vi "write.vi"() -> ()   [LabVIEW 2016]
uses:
  <vilib>/Instr/_visa.llb/VISA Configure Serial Port (Serial Instr).vi
panel:
  out "Numeric":dbl
  in  "Set Relay voltage":dbl(slide)=9.0 scale=0.0..10.0
  out "Compressor Status":bool
  out "Helium Underpressure":bool=TRUE
  in  "Pressure Lower Limit":dbl=0.1
  out "Helium Overpressure":bool
  in  "Pressure Upper Limit":dbl=2.8
  in  "Reading 2":string(combo)="255:R:OTEMP"
  out "Monitor 2":dbl(graph)
  out "Temperature":dbl=23.05
  in  "monitor 2 read length":u32=25
  out "monitor 2 feedback":string
  in  "Reading 1":string(combo)="255:R:MRMD"
  in  "Abort monitoring":bool
  out "Puressure":dbl=0.009
  in  "monitor 1 read length":u32=25
  out "Monitor 1":dbl(graph)
  out "Monitor 1 feedback":string
  # "psi"
  # "°C"
  # "Serial Port I/O control"
  # "Relay Configuration"
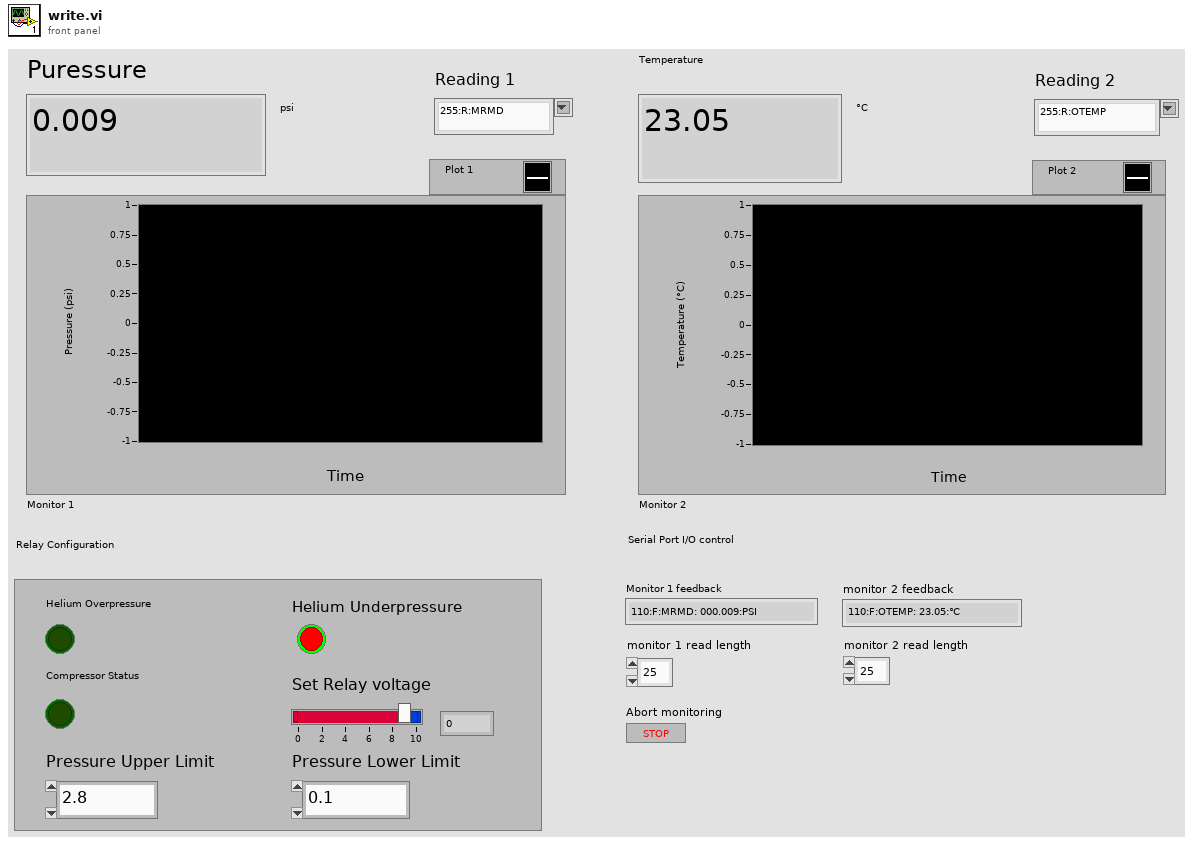
[diagram p1: front panel]
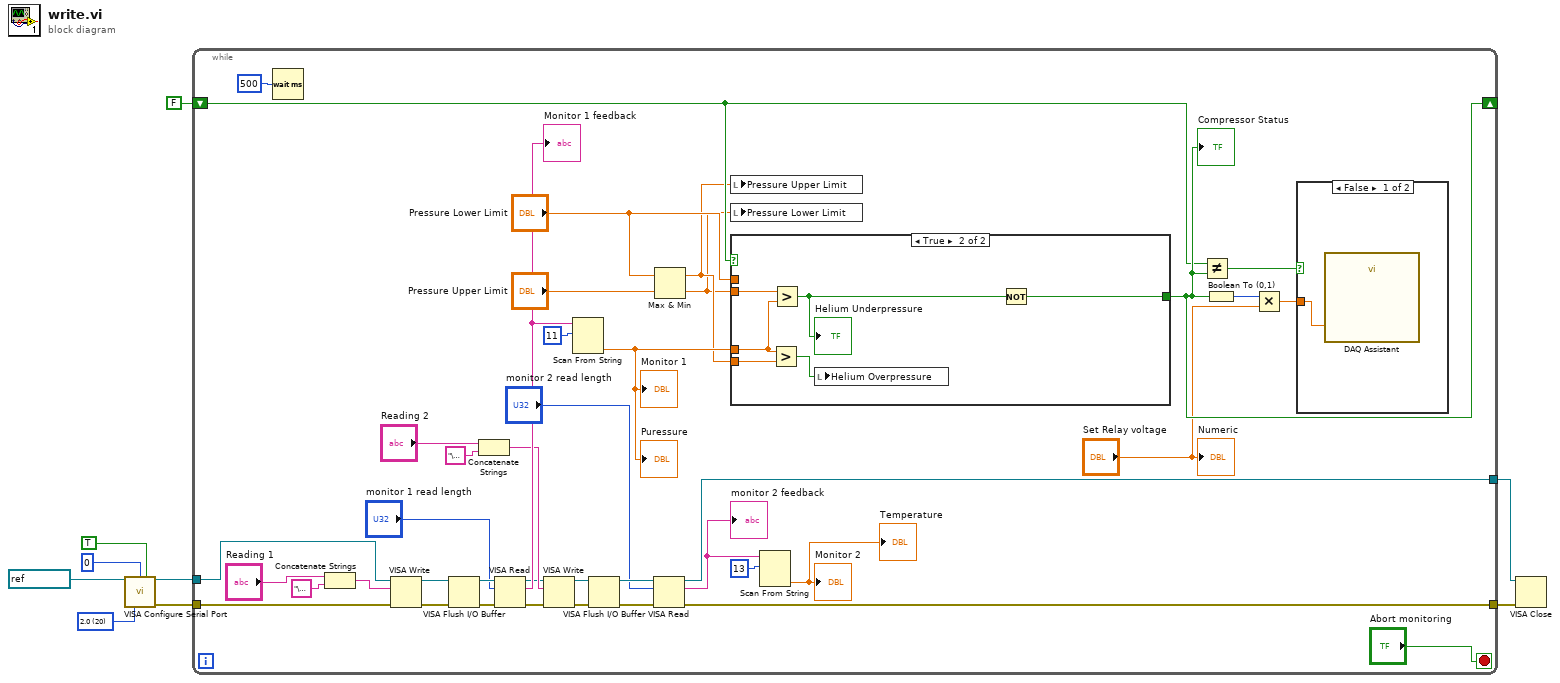
[diagram p0: block diagram]
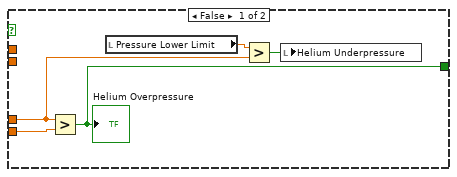
[diagram p3: hidden frame]
diagram:
  w4 = u16 20 items=["1.0"=10, "1.5"=15, "2.0"=20] ("stop bits (10: 1 bit)")
  n1 = call-poly "VISA Configure Serial Port"("VISA resource name"=refnum<visa-resource-name> "COM2", "termination char\n(0xA = '\\n' = LF)"=u8 0 ("termination char\n(0xA = '\\n' = LF)"), "Enable Termination\nChar (T)"=TRUE ("Enable Termination\nChar (T)"), "stop bits (10: 1 bit)"=w4) -> ("VISA resource name out"=w1:refnum<visa-resource-name>, "error out"=w3:errorcluster)  [unwired: 10 in]
  n2 = while {
    tunnel: [w23] -> w9
    tunnel: [w24] -> w8
    tunnel: w3 -> [w41]
    shift-right: [w19] -> _
    shift-left: FALSE -> [w18]
    tunnel: w1 -> [w12]
    stop <- "Abort monitoring" stop-if-true
    n3 = Wait (ms)(milliseconds to wait=u32 500) -> ()  [unwired: 1 out]
    n4 = Concatenate Strings("Reading 1", "\u0000") -> (w49:string)
    n5 = VISA Write(VISA resource name=w12, write buffer=w49, error in (no error)=w41) -> (VISA resource name out=w45:refnum<visa-resource-name>, error out=w47:errorcluster)  [unwired: 1 out]
    n6 = VISA Flush I/O Buffer(VISA resource name=w45, error in (no error)=w47) -> (VISA resource name out=w46:refnum<visa-resource-name>, error out=w40:errorcluster)  [unwired: 1 in]
    n7 = Concatenate Strings("Reading 2", "\u0000") -> (w36:string)
    n8 = VISA Read(VISA resource name=w46, byte count="monitor 1 read length", error in (no error)=w40) -> (VISA resource name out=w26:refnum<visa-resource-name>, read buffer=w43:string, error out=w25:errorcluster)  [unwired: 1 out]
    "Monitor 1 feedback" <- w43
    n9 = VISA Write(VISA resource name=w26, write buffer=w36, error in (no error)=w25) -> (VISA resource name out=w32:refnum<visa-resource-name>, error out=w34:errorcluster)  [unwired: 1 out]
    n10 = Scan From String(input string=w43, initial scan location=u32 11) -> (output 1=w22:dbl)  [unwired: 3 in, 3 out]
    "Puressure" <- w22
    "Monitor 1" <- w22
    n11 = VISA Flush I/O Buffer(VISA resource name=w32, error in (no error)=w34) -> (VISA resource name out=w33:refnum<visa-resource-name>, error out=w28:errorcluster)  [unwired: 1 in]
    n12 = VISA Read(VISA resource name=w33, byte count="monitor 2 read length", error in (no error)=w28) -> (VISA resource name out=w24:refnum<visa-resource-name>, read buffer=w30:string, error out=w23:errorcluster)  [unwired: 1 out]
    "monitor 2 feedback" <- w30
    n13 = Max & Min(x="Pressure Lower Limit", y="Pressure Upper Limit") -> (max(x,y)=w14:dbl, min(x,y)=w13:dbl)
    n14 = local write "Pressure Upper Limit"(w14) -> ()
    n15 = local write "Pressure Lower Limit"(w13) -> ()
    n16 = case shown="True" w18 {
      tunnel: w22 -> [w54 w60]
      tunnel: [w55 w58] -> w19
      tunnel: "Pressure Lower Limit" -> [_ _]
      tunnel: w14 -> [w51 w56]
      tunnel: w13 -> [_ w57]
      frame False {
        n17 = Greater?(x=w54, y=w51) -> (0:w55:bool)
        "Helium Overpressure" <- w55
        n18 = local read "Pressure Lower Limit"() -> (w53:dbl)
        n19 = Greater?(x=w53, y=w54) -> (0:w52:bool)
        n20 = local write "Helium Underpressure"(w52) -> ()
      }
      frame True {
        n21 = Greater?(x=w60, y=w56) -> (0:w61:bool)
        n22 = Greater?(x=w57, y=w60) -> (0:w59:bool)
        "Helium Underpressure" <- w59
        n23 = local write "Helium Overpressure"(w61) -> ()
        n24 = Not(x=w59) -> (.not. x?=w58:bool)
      }
    }
    "Compressor Status" <- w19
    n25 = Scan From String(input string=w30, initial scan location=u32 13) -> (output 1=→"Temperature" →"Monitor 2":dbl)  [unwired: 3 in, 3 out]
    n26 = Not Equal?(x=w18, y=w19) -> (x != y?=w17:bool)
    n27 = Boolean To (0,1)(Boolean=w19) -> (0, 1=w21:i16)
    n28 = Multiply(x=w21, y="Set Relay voltage") -> (x*y=w20:dbl)
    n29 = case shown="False" w17 {
      tunnel: w20 -> [w50 _]
      frame False {
        n30 = call "DAQ Assistant"("data"=w50) -> ()  [unwired: 17 in, 2 out]
      }
      frame True {
      }
    }
    "Numeric" <- "Set Relay voltage"
  }
  n31 = VISA Close(VISA resource name=w8, error in (no error)=w9) -> ()  [unwired: 1 out]
